vi "Remote Update.vi"(8 "error in":errorcluster, 11 "Value":dbl format="%#_13g") -> (0 "error out":errorcluster)   [LabVIEW 2015, in "PLC.lvlib"]
uses:
  PLC.lvlib
  support/Message Queue/Message Queue.lvlib
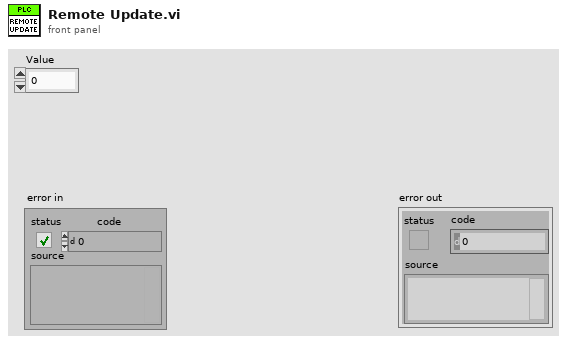
[diagram p1: front panel]
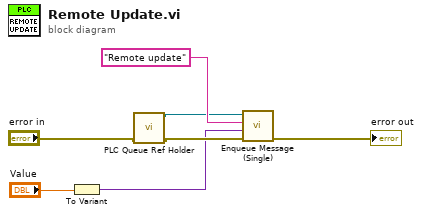
[diagram p0: block diagram]
diagram:
  n1 = To Variant(anything="Value") -> (Variant=w2:variant)
  n2 = call "PLC Queue Ref Holder.vi"("error in"="error in") -> ("error out"=w3:errorcluster, "Input Message Queue"=w4:refnum<queue>)  [unwired: 9 in]
  n3 = call "Enqueue Message (Single).vi"("error in (no error)"=w3, "Message Data"=w2, "Message"="Remote update", "Message Queue"=w4) -> ("error out"=→"error out":errorcluster)  [unwired: 6 in, 1 out]
